vi "from string.vi"(8 "error in":errorcluster, 9 "data":string, 10 "version":string, 11 "Standard Engine Repo Data in":refnum<class "Standard Engine Configuration.lvclass">) -> (0 "error out":errorcluster, 3 "Standard Engine Repo Data out":refnum<class "Standard Engine Configuration.lvclass">)   [LabVIEW 2013, in "Standard Engine Configuration.lvclass"]
uses:
  Standard Engine Configuration.lvclass
  timing policy.ctl
  <vilib>/NI/Module Execution Interface/Engine Configuration/engine configuration.lvclass
  Standard Engine Configuration.lvclass/Standard Engine Configuration.ctl
  Engine Configuration.ctl
  Loop Info.ctl
  Supported Timing Sources.ctl
  Module Specific Configuration.ctl
  Module Decimation.ctl
  Module Error Configuration.ctl
  Error Actions By Category.ctl
  <vilib>/NI/Tag Bus Module Framework/runtime/error classification.ctl
  Error Actions.ctl
  <vilib>/NI/Tag Bus Module Framework/root configuration/TBM configuration.lvclass
  <vilib>/NI/Tag Bus Module Framework/runtime/TBM module execution interface.lvclass
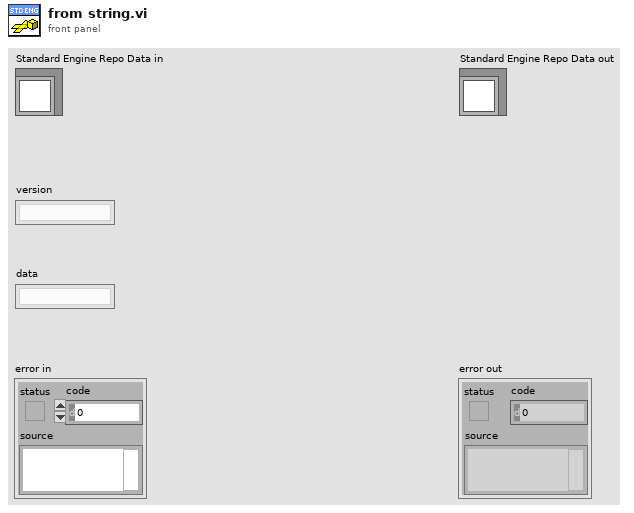
[diagram p1: front panel]
types:
  T1 = cluster{"Loop Info":cluster{"Processor":i32, "Priority":i32}, "Timing Source Type":enum16{"Use Module Timing Source", "1 kHz Clock", "1 MHz Clock", "Synchronize to Scan Engine"}, "Timing Source dt":u32, "Master Timing Module":string, "Module Specific Configuration":cluster{"Module ID":string, "Module Decimation":cluster{"Decimation":u16, "Offset":u16}, "Module Error Configuration":cluster{"Module Error Configuration":cluster{"error classification":enum16{"unknown", "none", "trivial", "recoverable", "critical"}, "Error Actions":enum16{"Clear", "Notify", "Stop Component", "Stop Engine", "Safe State", "Attempt Recovery"}[]}[]}, "execution order priority":i32, "async?":bool}[]}
  T2 = typedef "Standard Engine Configuration.lvclass/timing policy.ctl" = enum16{"strict determinism", "nonblocking", "nondeterministic inline"}
  T3 = typedef "Standard Engine Configuration.lvclass/Engine Configuration.ctl" = cluster{"Loop Info":T4, "Timing Source Type":T5, "Timing Source dt":u32, "Master Timing Module":string, "Module Specific Configuration":T6[]}
  T4 = typedef "Standard Engine Configuration.lvclass/Loop Info.ctl" = cluster{"Processor":i32, "Priority":i32}
  T5 = typedef "Standard Engine Configuration.lvclass/Supported Timing Sources.ctl" = enum16{"Use Module Timing Source", "1 kHz Clock", "1 MHz Clock", "Synchronize to Scan Engine"}
  T6 = typedef "Standard Engine Configuration.lvclass/Module Specific Configuration.ctl" = cluster{"Module ID":string, "Module Decimation":T7, "Module Error Configuration":T8, "execution order priority":i32, "async?":bool, "report error?":bool, "error tag":string}
  T7 = typedef "Standard Engine Configuration.lvclass/Module Decimation.ctl" = cluster{"Decimation":u16, "Offset":u16}
  T8 = typedef "Standard Engine Configuration.lvclass/Module Error Configuration.ctl" = cluster{"Module Error Configuration":T9[]}
  T9 = typedef "Standard Engine Configuration.lvclass/Error Actions By Category.ctl" = cluster{"error classification":T10, "Error Actions":T11[]}
  T10 = typedef "TBM module execution interface.lvclass/error classification.ctl" = enum16{"unknown", "none", "trivial", "recoverable", "critical"}
  T11 = typedef "Standard Engine Configuration.lvclass/Error Actions.ctl" = enum16{"Clear", "Notify", "Stop Component", "Stop Engine", "Safe State", "Attempt Recovery"}
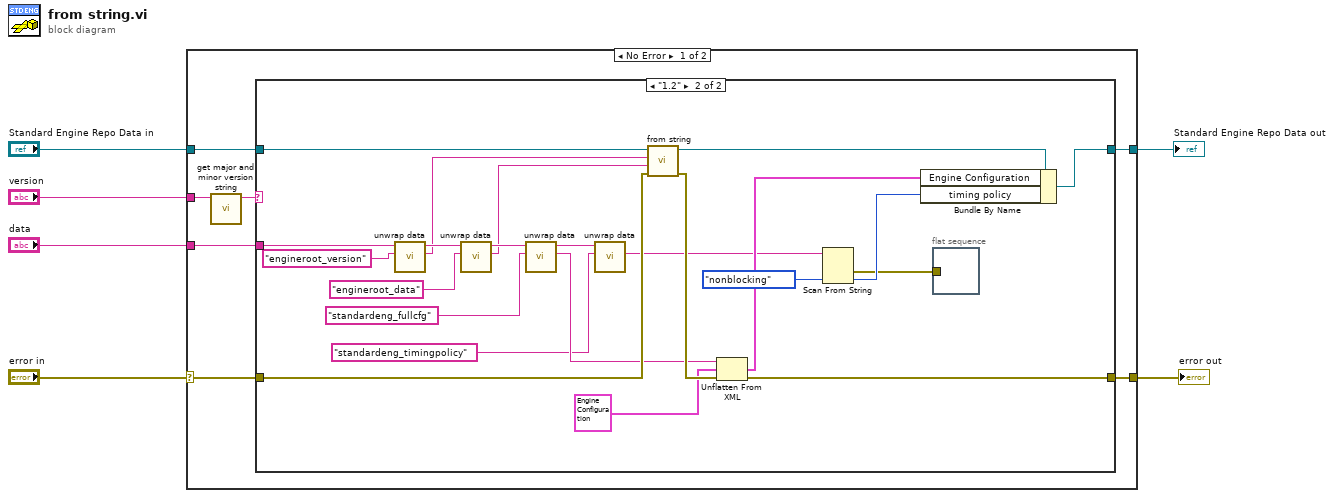
[diagram p0: block diagram]
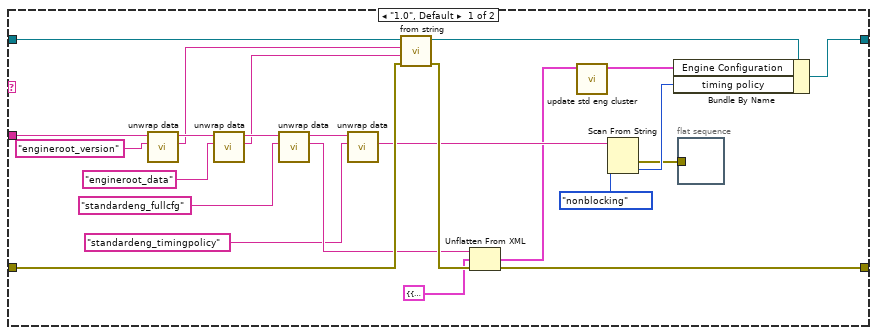
[diagram p2: hidden frame]
diagram:
  n1 = case shown="No Error" "error in" {
    selector: "error in" -> [w7 w61]
    tunnel: [w13 w61] -> w6
    tunnel: [w12 w62] -> w5
    tunnel: "data" -> [w11 _]
    tunnel: "Standard Engine Repo Data in" -> [w10 w62]
    tunnel: "version" -> [w9 _]
    frame No Error {
      n2 = call <vilib>:"get major and minor version string.vi"("full version"=w9) -> ("major.minor version"=w8:string)  [unwired: 10 in]
      n3 = case shown="\"1.2\"" w8 {
        tunnel: w7 -> [w37 w60]
        tunnel: [w32 w55] -> w13
        tunnel: [w35 w58] -> w12
        tunnel: w11 -> [w26 w48]
        tunnel: w10 -> [w34 w57]
        frame "1.0", Default {
          n4 = call <vilib>:"unwrap data.vi"("identifier"="engineroot_version" ("additional identifier"), "data to unwrap"=w26) -> ("unwrapped data"=w25:string, "remaining string"=w27:string)  [unwired: 8 in]
          n5 = call <vilib>:"unwrap data.vi"("identifier"="engineroot_data" ("additional identifier"), "data to unwrap"=w27) -> ("unwrapped data"=w23:string, "remaining string"=w30:string)  [unwired: 8 in]
          n6 = call <vilib>:"unwrap data.vi"("identifier"="standardeng_fullcfg" ("additional identifier"), "data to unwrap"=w30) -> ("unwrapped data"=w24:string, "remaining string"=w22:string)  [unwired: 8 in]
          n7 = call <vilib>:"unwrap data.vi"("identifier"="standardeng_timingpolicy" ("additional identifier"), "data to unwrap"=w22) -> ("unwrapped data"=w20:string)  [unwired: 8 in, 1 out]
          n8 = call-parent "from string.vi"("error in"=w37, "data"=w23, "version"=w25, "engine configuration in"=w34) -> ("error out"=w36:errorcluster, "engine configuration out"=w33:refnum<class "Standard Engine Configuration.lvclass">)  [unwired: 6 in]
          n9 = Unflatten From XML(xml string=w24, type=T1 {"Loop Info"={"Processor"=0, "Priority"=0}, "Timing Source Type"=enum."Use Module Timing Source", "Timing Source dt"=0, "Master Timing Module"="", "Module Specific Configuration"=[]} ("Engine Configuration"), error in (no error)=w36) -> (value=w14:T1, error out=w32:errorcluster)
          n10 = call "update std eng cluster.vi"("Engine Configuration in"=w14) -> ("Engine Configuration out"=w15:T3)  [unwired: 10 in]
          n11 = Scan From String(input string=w20, default 1=timing_policy."nonblocking" ("timing policy")) -> (error out=w17:errorcluster, output 1=w18:T2)  [unwired: 3 in, 2 out]
          n12 = Bundle By Name(cluster=w33, "Engine Configuration"=w15, "timing policy"=w18) -> (w35:refnum<class "Standard Engine Configuration.lvclass">)
          n13 = flat-sequence {
            tunnel: w17 -> [_]
            frame #0 {
            }
          }
        }
        frame "1.2" {
          n14 = call <vilib>:"unwrap data.vi"("identifier"="engineroot_version" ("additional identifier"), "data to unwrap"=w48) -> ("unwrapped data"=w47:string, "remaining string"=w49:string)  [unwired: 8 in]
          n15 = call <vilib>:"unwrap data.vi"("identifier"="engineroot_data" ("additional identifier"), "data to unwrap"=w49) -> ("unwrapped data"=w45:string, "remaining string"=w52:string)  [unwired: 8 in]
          n16 = call <vilib>:"unwrap data.vi"("identifier"="standardeng_fullcfg" ("additional identifier"), "data to unwrap"=w52) -> ("unwrapped data"=w46:string, "remaining string"=w44:string)  [unwired: 8 in]
          n17 = call <vilib>:"unwrap data.vi"("identifier"="standardeng_timingpolicy" ("additional identifier"), "data to unwrap"=w44) -> ("unwrapped data"=w42:string)  [unwired: 8 in, 1 out]
          n18 = call-parent "from string.vi"("error in"=w60, "data"=w45, "version"=w47, "engine configuration in"=w57) -> ("error out"=w59:errorcluster, "engine configuration out"=w56:refnum<class "Standard Engine Configuration.lvclass">)  [unwired: 6 in]
          n19 = Unflatten From XML(xml string=w46, type=T3 {"Loop Info"={"Processor"=0, "Priority"=0}, "Timing Source Type"=enum."Use Module Timing Source", "Timing Source dt"=0, "Master Timing Module"="", "Module Specific Configuration"=[]} ("Engine Configuration"), error in (no error)=w59) -> (value=w54:T3, error out=w55:errorcluster)
          n20 = Scan From String(input string=w42, default 1=timing_policy."nonblocking" ("timing policy")) -> (error out=w39:errorcluster, output 1=w40:T2)  [unwired: 3 in, 2 out]
          n21 = Bundle By Name(cluster=w56, "Engine Configuration"=w54, "timing policy"=w40) -> (w58:refnum<class "Standard Engine Configuration.lvclass">)
          n22 = flat-sequence {
            tunnel: w39 -> [_]
            frame #0 {
            }
          }
        }
      }
    }
    frame Error {
    }
  }
  "error out" <- w6
  "Standard Engine Repo Data out" <- w5
